vi "Calculate Satellite Relative Position.vi"(11 "Angle [deg]":sgl) -> (3 "Position":refnum<class "Vector 2D.lvclass">)   [LabVIEW 2021, in "Chmmr.lvclass"]
uses:
  Chmmr.lvclass
  Vector 2D/Vector 2D.lvclass
panel:
  in  "Radius":sgl=60.0
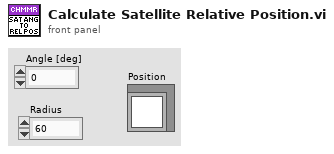
[diagram p1: front panel]
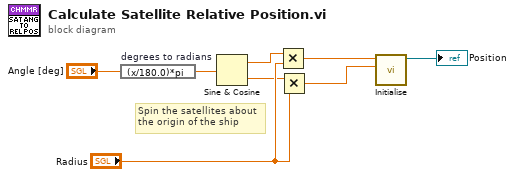
[diagram p0: block diagram]
diagram:
  # "Spin the satellites about the origin of the ship"
  n1 = expression code="(x/180.0)*pi" "degrees to radians"("Angle [deg]") -> (w5:sgl)
  n2 = Sine & Cosine(0:w5) -> (1:w7:sgl, 2:w6:sgl)
  n3 = Multiply(x=w7, y="Radius") -> (x*y=w3:sgl)
  n4 = Multiply(x=w6, y="Radius") -> (x*y=w2:sgl)
  n5 = call "Initialise.vi"("y"=w2, "x"=w3) -> ("Vector 2D out"=→"Position":refnum<class "Vector 2D.lvclass">)  [unwired: 9 in]
